vi "Gear Mechanism.vi"(0 "gearServo":string="gearServo", 1 "Angle 1":dbl, 2 "Angle 2":dbl, 3 "Button 1":bool, 4 "Button 2":bool, 5 "error in":errorcluster) -> (19 "error out":errorcluster)   [LabVIEW 2016]
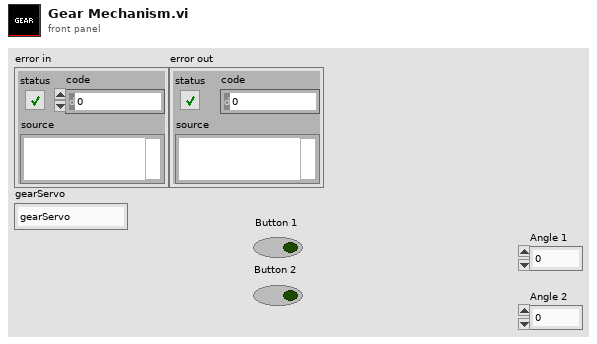
[diagram p1: front panel]
types:
  T1 = typedef "WPI_ServoDeviceRef.ctl" = cluster{"DeviceStatus":errorcluster, "PWM Channel":T2, "DeadBand":T3}
  T2 = typedef "FPGA_DIOPWMChannel.ctl" = enum8{"PWM 0", "PWM 1", "PWM 2", "PWM 3", "PWM 4", "PWM 5", "PWM 6", "PWM 7", "PWM 8", "PWM 9", "PWM MXP 0", "PWM MXP 1", "PWM MXP 2", "PWM MXP 3", "PWM MXP 4", "PWM MXP 5", "PWM MXP 6", "PWM MXP 7", "PWM MXP 8", "PWM MXP 9", "Invalid"}
  T3 = typedef "WPI_PWMDeadband.ctl" = cluster{"Name":string, "maxPositivePwm":i32, "minPositivePwm":i32, "centerPwm":i32, "maxNegativePwm":i32, "minNegativePwm":i32, "angularRange":u16}
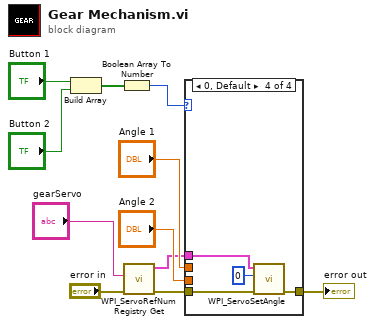
[diagram p0: block diagram]
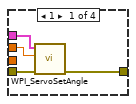
[diagram p2: hidden frame]
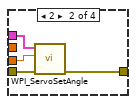
[diagram p3: hidden frame]
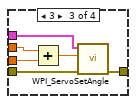
[diagram p4: hidden frame]
diagram:
  n1 = Build Array("Button 1", "Button 2") -> (w7:bool[])
  n2 = Boolean Array To Number(Boolean array=w7) -> (number=w6:u32)
  n3 = call <vilib>:"WPI_ServoRefNum Registry Get.vi"("error in (no error)"="error in", "refnum name"="gearServo") -> ("error out"=w2:errorcluster, "ServoDeviceRef"=w4:T1)  [unwired: 8 in]
  n4 = case shown="0, Default" w6 {
    tunnel: w4 -> [w15 w19 w25 w29]
    tunnel: "Angle 1" -> [w14 _ w24 _]
    tunnel: "Angle 2" -> [_ w18 w23 _]
    tunnel: [w13 w16 w20 w27] -> w5
    tunnel: w2 -> [w12 w17 w21 w28]
    frame 1 {
      n5 = call <vilib>:"WPI_ServoSetAngle.vi"("error in (no error)"=w12, "Angle"=w14, "ServoDeviceRef"=w15) -> ("error out"=w13:errorcluster)  [unwired: 7 in, 1 out]
    }
    frame 2 {
      n6 = call <vilib>:"WPI_ServoSetAngle.vi"("error in (no error)"=w17, "Angle"=w18, "ServoDeviceRef"=w19) -> ("error out"=w16:errorcluster)  [unwired: 7 in, 1 out]
    }
    frame 3 {
      n7 = Add(x=w24, y=w23) -> (x+y=w22:dbl)
      n8 = call <vilib>:"WPI_ServoSetAngle.vi"("error in (no error)"=w21, "Angle"=w22, "ServoDeviceRef"=w25) -> ("error out"=w20:errorcluster)  [unwired: 7 in, 1 out]
    }
    frame 0, Default {
      n9 = call <vilib>:"WPI_ServoSetAngle.vi"("error in (no error)"=w28, "Angle"=0, "ServoDeviceRef"=w29) -> ("error out"=w27:errorcluster)  [unwired: 7 in, 1 out]
    }
  }
  "error out" <- w5
